vi "Destroy Image Window.vi"(8 "error in (no error)":errorcluster, 10 "Window Name":string) -> (0 "error out":errorcluster, 2 "Already Closed":bool)   [LabVIEW 2020, in "g_ar_toolkit.lvlib"]
uses:
  g_ar_toolkit.lvlib
  g_ar_toolkit.32.dll
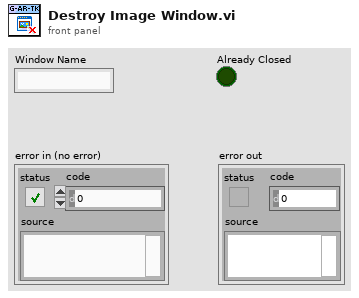
[diagram p1: front panel]
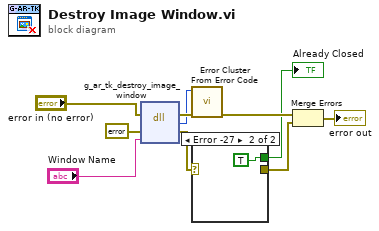
[diagram p0: block diagram]
diagram:
  n1 = dll-call lib="C:/serenial/libraries/g-augmented-reality-toolkit/LabVIEW/g_ar_toolkit/g_ar_toolkit.*.*" fn="g_ar_tk_destroy_image_window"(error in="error in (no error)", "error_cluster"=errorcluster {"status"=FALSE, "code"=0, "source"=""} ("error constant"), "window_name"="Window Name") -> (error out=w10:errorcluster, "MgErr"=w9:i32, "error_cluster"=w3:errorcluster)  [unwired: 3 in, 1 out]
  n2 = call <vilib>:"Error Cluster From Error Code.vi"("error in (no error)"=w10, "error code (0)"=w9) -> ("error out"=w8:errorcluster)  [unwired: 7 in]
  n3 = case shown="Error -27" w3 {
    selector: w3 -> [w11 _]
    tunnel: [w11 _] -> w2
    tunnel: [_ TRUE] -> w1
    frame #0 {
    }
    frame #1 {
    }
  }
  "Already Closed" <- w1
  n4 = Merge Errors(w8, w2) -> (→"error out":errorcluster)
